vi "loadCRHSocketReportYield.vi"() -> ()   [LabVIEW 2012]
uses:
  <vilib>/addons/database/Connection.llb/DB Tools Open Connec (Path).vi
  <vilib>/addons/database/Connection.llb/Conn Execute.vi
  <vilib>/addons/database/Recordset.llb/Rec Destroy - Connection.vi
  <vilib>/addons/database/NI_Database_API.lvlib
panel:
  out "error out":errorcluster
  out "concatenated string":string
  out "after substring":string
  out "after substring 2":string
  out "String":string
  out "array":string[][](array[string])
  in  "path":path=path "C:/temp/SocketReport"
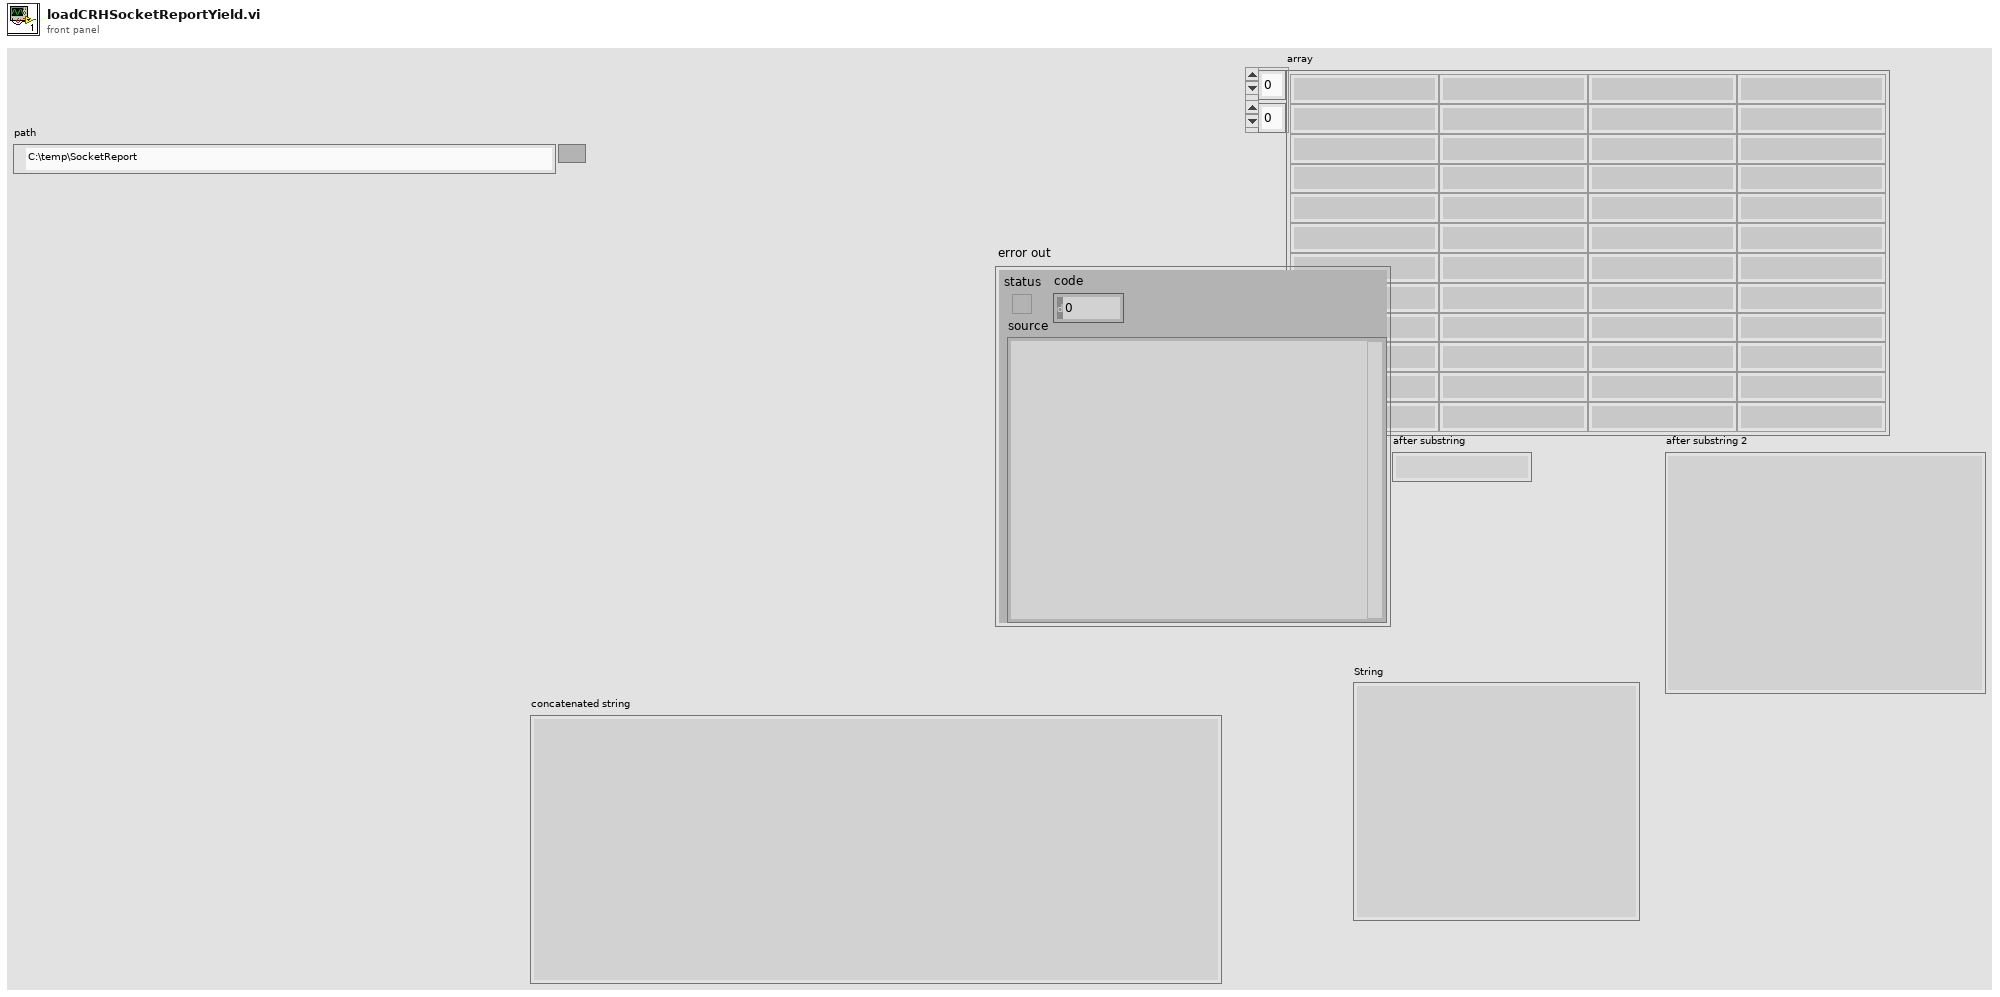
[diagram p1: front panel]
types:
  T1 = typedef "NI_Database_API.lvlib/Conn ObjectReference.ctl" = refnum<k1>
  T2 = typedef "NI_Database_API.lvlib/Rec ObjectReference.ctl" = refnum<k1>
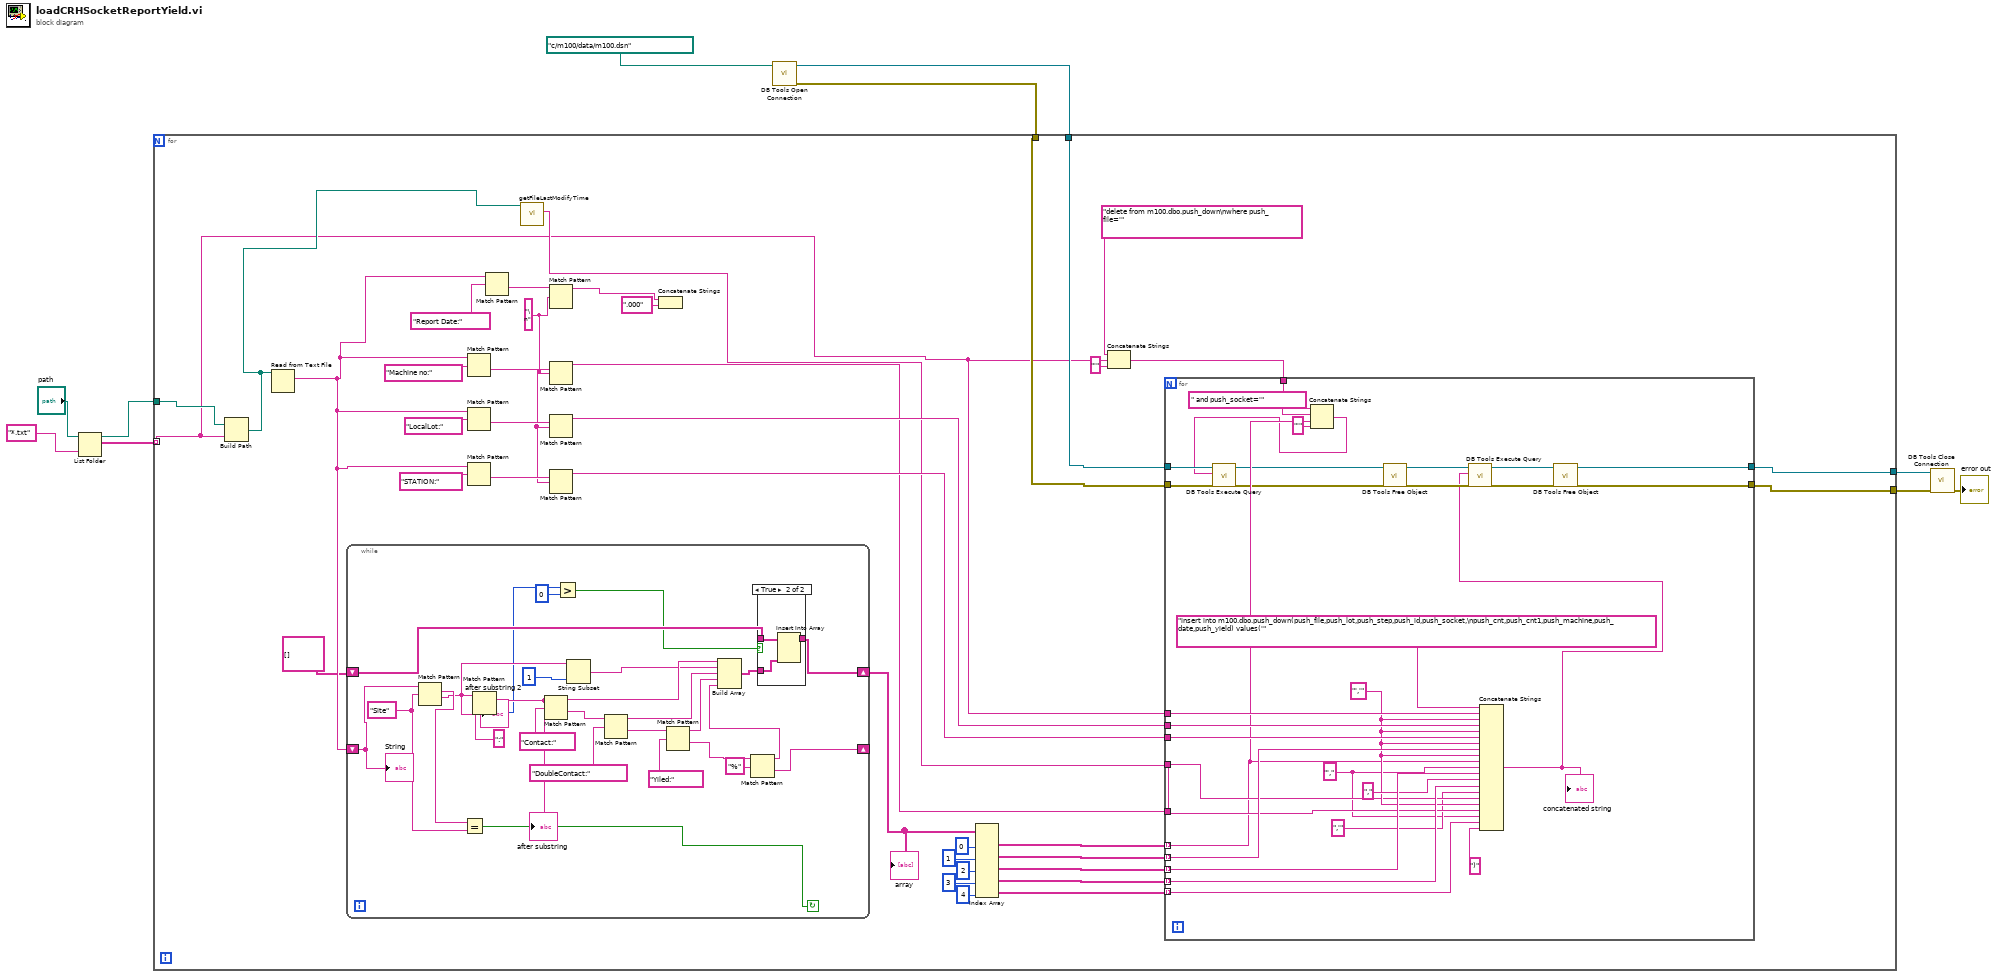
[diagram p0: block diagram]
diagram:
  n1 = List Folder(path="path", pattern="*.txt") -> (path out=w8:path, filenames=w1:string[])  [unwired: 2 in, 2 out]
  n2 = call-poly <vilib>:"DB Tools Open Connection.vi"("connection information"=path "c:/m100/data/m100.dsn") -> ("error out"=w2:errorcluster, "connection reference"=w3:T1)  [unwired: 7 in]
  n3 = for {
    tunnel: w8 -> [w15]
    tunnel: [w19] -> w6
    tunnel: [w18] -> w5
    tunnel: w3 -> [w17]
    tunnel: w2 -> [w16]
    tunnel: w1 -> [w13] mode=indexing
    w38 = "\n" ("regular expression")
    n4 = Build Path(base path=w15, name or relative path=w13) -> (appended path=w14:path)
    n5 = Read from Text File(file (use dialog)=w14) -> (text=w23:string)  [unwired: 3 in, 3 out]
    n6 = while {
      shift-right: [w51] -> _
      shift-left: w23 -> [w64]
      shift-right: [w63] -> w21
      shift-left: string[][] [] ("array") -> [w62]
      stop <- w59 continue-if-true
      w60 = "Site" ("regular expression")
      n7 = Match Pattern(string=w64, regular expression=w60) -> (match substring=w61:string, after substring=w56:string)  [unwired: 1 in, 2 out]
      "after substring 2" <- w56
      n8 = Equal?(x=w61, y=w60) -> (x = y?=w59:bool)
      n9 = Match Pattern(string=w56, regular expression=":") -> (after substring=w58:string, offset past match=w55:i32)  [unwired: 1 in, 2 out]
      "after substring" <- w58
      n10 = Match Pattern(string=w58, regular expression="Contact:") -> (before substring=w74:string, after substring=w72:string)  [unwired: 1 in, 2 out]
      n11 = Greater?(x=w55, y=0) -> (0:w53:bool)
      n12 = String Subset(string=w56, length (rest)=1 ("length (rest)")) -> (substring=w65:string)  [unwired: 1 in]
      n13 = Match Pattern(string=w72, regular expression="DoubleContact:") -> (before substring=w68:string, after substring=w70:string)  [unwired: 1 in, 2 out]
      n14 = Match Pattern(string=w70, regular expression="Yiled:") -> (before substring=w67:string, after substring=w52:string)  [unwired: 1 in, 2 out]
      n15 = Match Pattern(string=w52, regular expression="%") -> (before substring=w49:string, after substring=w51:string)  [unwired: 1 in, 2 out]
      n16 = Build Array(w74, w65, w68, w67, w49) -> (w73:string[])
      n17 = case shown="True" w53 {
        tunnel: w73 -> [_ w79]
        tunnel: [w76 w78] -> w63
        tunnel: w62 -> [w76 w77]
        frame False {
        }
        frame True {
          n18 = Insert Into Array(array=w77, new element=w79) -> (w78:string[][])  [unwired: 2 in]
        }
      }
      "String" <- w64
    }
    "array" <- w21
    n19 = Match Pattern(string=w23, regular expression="Machine no:") -> (after substring=w47:string)  [unwired: 1 in, 3 out]
    n20 = Match Pattern(string=w23, regular expression="LocalLot:") -> (after substring=w41:string)  [unwired: 1 in, 3 out]
    n21 = Match Pattern(string=w23, regular expression="STATION:") -> (after substring=w39:string)  [unwired: 1 in, 3 out]
    n22 = Match Pattern(string=w23, regular expression="Report Date:") -> (after substring=w43:string)  [unwired: 1 in, 3 out]
    n23 = call "getFileLastModifyTime.vi"("path"=w14) -> ("date/time string"=w20:string)  [unwired: 10 in]
    n24 = Match Pattern(string=w43, regular expression=w38) -> (before substring=w26:string)  [unwired: 1 in, 3 out]
    n25 = Match Pattern(string=w47, regular expression=w38) -> (before substring=w24:string)  [unwired: 1 in, 3 out]
    n26 = Match Pattern(string=w41, regular expression=w38) -> (before substring=w34:string)  [unwired: 1 in, 3 out]
    n27 = Match Pattern(string=w39, regular expression=w38) -> (before substring=w33:string)  [unwired: 1 in, 3 out]
    n28 = Concatenate Strings(w26, ".000" ("string")) -> ()  [unwired: 1 out]
    n29 = Index Array(array=w21, index (col) #1=0 ("disabled index (col)"), index (col) #2=1 ("index (col)"), index (col) #3=2 ("index (col)"), index (col) #4=3 ("index (col)"), index (col) #5=4 ("index (col)")) -> (element #1=w29:string[], element #2=w30:string[], element #3=w28:string[], element #4=w27:string[], element #5=w11:string[])  [unwired: 5 in]
    n30 = Concatenate Strings("delete from m100.dbo.push_down\nwhere push_file='", w13, "'" ("string")) -> (w35:string)
    n31 = for {
      tunnel: w17 -> [w110]
      tunnel: [w108] -> w19
      tunnel: w16 -> [w107]
      tunnel: [w105] -> w18
      tunnel: w35 -> [w93]
      tunnel: w13 -> [w103]
      tunnel: w34 -> [w102]
      tunnel: w33 -> [w101]
      tunnel: w30 -> [w100] mode=indexing
      tunnel: w29 -> [w91] mode=indexing
      tunnel: w28 -> [w99] mode=indexing
      tunnel: w27 -> [w97] mode=indexing
      tunnel: w20 -> [w96]
      tunnel: w24 -> [w94]
      tunnel: w11 -> [w81] mode=indexing
      w80 = "'," ("string")
      w95 = "','" ("string")
      n32 = Concatenate Strings(w93, " and push_socket='" ("string"), w91, "'" ("string")) -> (w89:string)
      n33 = call-poly <vilib>:"DB Tools Execute Query.vi"("error in (no error)"=w107, "SQL query"=w89, "connection reference"=w110) -> ("error out"=w84:errorcluster, "recordset reference"=w85:T2)  [unwired: 5 in]
      n34 = call-poly <vilib>:"DB Tools Free Object.vi"("error in (no error)"=w84, "recordset reference"=w85) -> ("error out"=w106:errorcluster, "connection reference"=w109:T1)  [unwired: 8 in]
      n35 = Concatenate Strings("insert into m100.dbo.push_down(push_file,push_lot,push_step,push_id,push_socket,\npush_cnt,push_cnt1,push_machine,push_date,push_yield) values('", w103, w95, w102, w95, w101, w95, w100, w95, w91, w80, w99, "," ("string"), w97, ",'" ("string"), w94, w95, w96, w80, w81, ")" ("string")) -> (w88:string)
      "concatenated string" <- w88
      n36 = call-poly <vilib>:"DB Tools Execute Query.vi"("error in (no error)"=w106, "SQL query"=w88, "connection reference"=w109) -> ("error out"=w86:errorcluster, "recordset reference"=w87:T2)  [unwired: 5 in]
      n37 = call-poly <vilib>:"DB Tools Free Object.vi"("error in (no error)"=w86, "recordset reference"=w87) -> ("error out"=w105:errorcluster, "connection reference"=w108:T1)  [unwired: 8 in]
    }
  }
  n38 = call <vilib>:"DB Tools Close Connection.vi"("error in (no error)"=w5, "connection reference"=w6) -> ("error out"=→"error out":errorcluster)  [unwired: 5 in]
